vi "fakeImFromScanSettingsForTest.vi"(11 "scan specification":T1={"x amplitude"=100, "x resolution (pixels)"=28, "x offset fly-forward (iterations)"=50, "x offset fly-back (iterations)"=100, "y resolution (nr. of lines)"=80, "y step size"=30, "iterations per pixel"=5, "number of frames"=80, "y offset (pixels)"=0, "number of y-brake lines  (before y-fly-back)"=0, "number y-brake lines (after y-fly-back)"=40, "number of y-fly-back steps"=0, "lines per z step"=1, "number of z/intensity tuples"=228, "number of repetitions (volumes or planes)"=1000, "z step size derived"=32, "choose the beginning of z scan"=FALSE, "number of frames (settings)"=80, "FPGA trajectory?"=TRUE, "Pockels cell voltage (bits)"=0, "Vy min(bits)"=0, "Vz min(bits)"=0}) -> (3 "fake 2 ch im":u32[](array[numeric]))   [LabVIEW 2010]
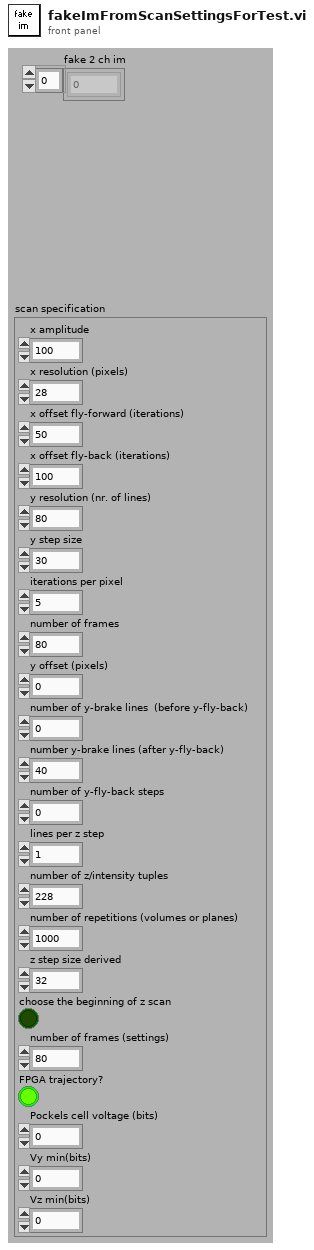
[diagram p1: front panel]
types:
  T1 = cluster{"x amplitude":u16, "x resolution (pixels)":u16, "x offset fly-forward (iterations)":u16, "x offset fly-back (iterations)":u16, "y resolution (nr. of lines)":u16, "y step size":u16, "iterations per pixel":u16, "number of frames":i32, "y offset (pixels)":u16, "number of y-brake lines  (before y-fly-back)":u16, "number y-brake lines (after y-fly-back)":u16, "number of y-fly-back steps":u16, "lines per z step":u16, "number of z/intensity tuples":u16, "number of repetitions (volumes or planes)":i32, "z step size derived":u16, "choose the beginning of z scan":bool, "number of frames (settings)":i32, "FPGA trajectory?":bool, "Pockels cell voltage (bits)":i16, "Vy min(bits)":i16, "Vz min(bits)":i16}
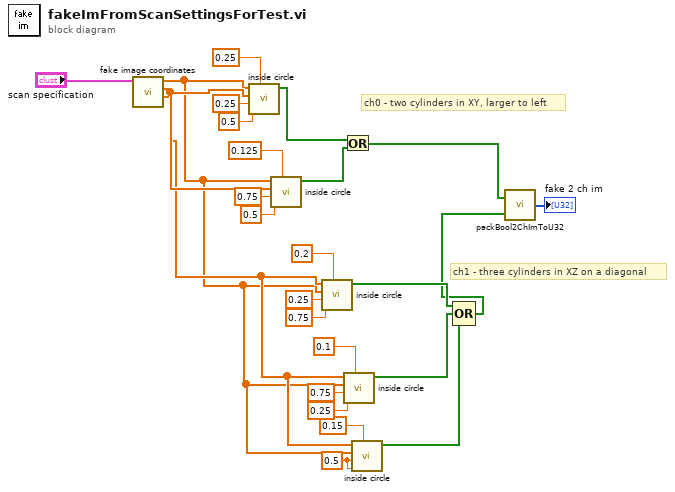
[diagram p0: block diagram]
diagram:
  w9 = 0.5 ("xc")
  # "ch1 - three cylinders in XZ on a diagonal"
  # "ch0 - two cylinders in XY, larger to left"
  n1 = call "fake image coordinates.vi"("scan specification"="scan specification") -> ("zcoords"=w11:dbl[], "ycoords"=w20:dbl[], "xcoords"=w10:dbl[])  [unwired: 8 in]
  n2 = call "inside circle.vi"("r"=0.25, "yc"=0.5, "xc"=0.25, "ycoords"=w20, "xcoords"=w10) -> ("inside circle"=w19:bool[])  [unwired: 6 in]
  n3 = call "inside circle.vi"("r"=0.125, "yc"=0.5, "xc"=0.75, "ycoords"=w20, "xcoords"=w10) -> ("inside circle"=w18:bool[])  [unwired: 6 in]
  n4 = call "inside circle.vi"("r"=0.2, "yc"=0.75, "xc"=0.25, "ycoords"=w10, "xcoords"=w11) -> ("inside circle"=w7:bool[])  [unwired: 6 in]
  n5 = Or(x=w19, y=w18) -> (x .or. y?=w4:bool[])
  n6 = call "inside circle.vi"("r"=0.1, "yc"=0.25, "xc"=0.75, "ycoords"=w10, "xcoords"=w11) -> ("inside circle"=w6:bool[])  [unwired: 6 in]
  n7 = call "inside circle.vi"("r"=0.15, "yc"=w9, "xc"=w9, "ycoords"=w10, "xcoords"=w11) -> ("inside circle"=w5:bool[])  [unwired: 6 in]
  n8 = Compound Arithmetic op=OR(w7, w6, w5) -> (w3:bool[])
  n9 = call "packBool2ChImToU32.vi"("ch1"=w3, "ch0"=w4) -> ("buffer"=→"fake 2 ch im":u32[])
